vi "config_test2.vi"() -> ()   [LabVIEW 2015]
uses:
  <vilib>/Utility/Data Type/NI_Data Type.lvlib
  <vilib>/Utility/config.llb/NI_LVConfig.lvlib
  <vilib>/Utility/config.llb/Write Key (I32).vi
  <vilib>/Utility/config.llb/Write Key (String).vi
  <vilib>/Utility/config.llb/Write Key (Double).vi
panel:
  in  "Tab Control":enum32{"Page 1", "Page 2"}(tab)
  in  "x":dbl
  in  "y":dbl
  out "x+y":dbl
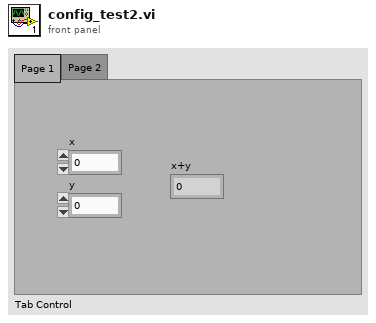
[diagram p1: front panel]
types:
  T1 = typedef "NI_LVConfig.lvlib/Config Data RefNum.ctl" = refnum<k1>
  T2 = typedef "NI_Data Type.lvlib/Data Type.ctl" = enum8{"Invalid Type", "Void", "I8", "I16", "I32", "I64", "U8", "U16", "U32", "U64", "Single Float", "Double Float", "Extended Float", "Single Complex", "Double Complex", "Extended Complex", "Enum U8", "Enum U16", "Enum U32", "Enum U64", "Single Float With Unit", "Double Float With Unit", "Extended Float With Unit", "Single Complex with Unit", "Double Complex with Unit", "Extended Complex with Unit", "Boolean", "String", "Path", "Picture", "Tag", "Array", "Cluster", "Variant", "LV Variant", "Waveform", "Timestamp", "Digital Waveform", "Digital Data", "ExpressData", "Refnum", "External Data", "VI", "Poly VI", "LabVIEW Class Instance", "Fixed Point"}
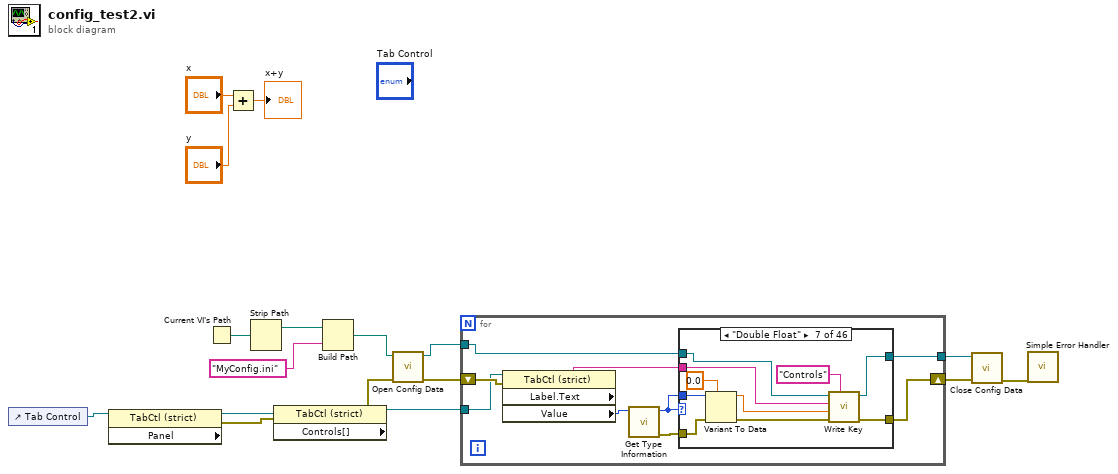
[diagram p0: block diagram]
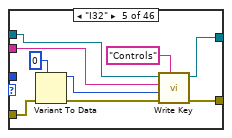
[diagram p6: hidden frame]
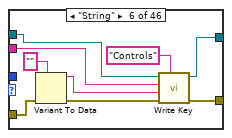
[diagram p7: hidden frame]
diagram:
  n1 = control-ref of="Tab Control"() -> (w14:refnum<vi>)
  n2 = property class="TabCtl (strict)" props=["Panel"](reference=w14) -> (reference out=w2:refnum<vi>, error out=w13:errorcluster)  [unwired: 1 in, 1 out]
  n3 = Current VI's Path() -> (path=w12:path)
  n4 = Add(x="x", y="y") -> (x+y=→"x+y":dbl)
  n5 = Strip Path(path=w12) -> (stripped path=w11:path)  [unwired: 1 out]
  n6 = property class="TabCtl (strict)" props=["Controls[]"](reference=w2, error in=w13) -> (reference out=w1:refnum<vi>, error out=w4:errorcluster)  [unwired: 1 out]
  n7 = Build Path(base path=w11, name or relative path="MyConfig.ini") -> (appended path=w9:path)
  n8 = call <vilib>:"Open Config Data.vi"("error in (no error)"=w4, "configuration file path"=w9) -> ("error out"=w3:errorcluster, "refnum"=w8:T1)  [unwired: 7 in, 1 out]
  n9 = for {
    tunnel: w8 -> [w22]
    shift-right: [w20] -> w6
    shift-left: w3 -> [w26]
    tunnel: [w21] -> w7
    tunnel: w1 -> [w19]
    n10 = property class="TabCtl (strict)"(reference=w19, error in=w26) -> ("Label.Text"=w23:string, "Value"=w24:enum32{"Page 1", "Page 2"})  [unwired: 2 out]
    n11 = call <vilib>:"Get Type Information.vi"("Variant"=w24) -> ("error out"=w25:errorcluster, "Type"=w18:T2)  [unwired: 6 in, 3 out]
    n12 = case shown="\"Double Float\"" w18 {
      tunnel: w25 -> [w27 w29 w31 w33 w43 w52 w62 w63 w65 w67 w69 w71 w73 w75 w77 w79 w81 w83 w85 w87 w89 w91 w93 w95 w97 w99 w101 w103 w105 w107 w109 w111 w113 w115 w117 w119 w121 w123 w125 w127 w129 w131 w133 w135 w137 w139]
      tunnel: w23 -> [_ _ _ _ w40 w49 w59 _ _ _ _ _ _ _ _ _ _ _ _ _ _ _ _ _ _ _ _ _ _ _ _ _ _ _ _ _ _ _ _ _ _ _ _ _ _ _]
      tunnel: w22 -> [w28 w30 w32 w34 w39 w48 w58 w64 w66 w68 w70 w72 w74 w76 w78 w80 w82 w84 w86 w88 w90 w92 w94 w96 w98 w100 w102 w104 w106 w108 w110 w112 w114 w116 w118 w120 w122 w124 w126 w128 w130 w132 w134 w136 w138 w140]
      tunnel: [w28 w30 w32 w34 w37 w46 w56 w64 w66 w68 w70 w72 w74 w76 w78 w80 w82 w84 w86 w88 w90 w92 w94 w96 w98 w100 w102 w104 w106 w108 w110 w112 w114 w116 w118 w120 w122 w124 w126 w128 w130 w132 w134 w136 w138 w140] -> w21
      tunnel: [w27 w29 w31 w33 w36 w45 w55 w63 w65 w67 w69 w71 w73 w75 w77 w79 w81 w83 w85 w87 w89 w91 w93 w95 w97 w99 w101 w103 w105 w107 w109 w111 w113 w115 w117 w119 w121 w123 w125 w127 w129 w131 w133 w135 w137 w139] -> w20
      tunnel: w18 -> [_ _ _ _ _ _ w53 _ _ _ _ _ _ _ _ _ _ _ _ _ _ _ _ _ _ _ _ _ _ _ _ _ _ _ _ _ _ _ _ _ _ _ _ _ _ _]
      frame "Invalid Type", Default {
      }
      frame "Void" {
      }
      frame "I8" {
      }
      frame "I16" {
      }
      frame "I32" {
        n13 = Variant To Data(error in=w43, type=0) -> (data=w41:i32, error out=w42:errorcluster)  [unwired: 1 in]
        n14 = call-poly <vilib>:"Write Key.vi"("section"="Controls", "error in (no error)"=w42, "value"=w41, "key"=w40, "refnum"=w39) -> ("error out"=w36:errorcluster, "refnum out"=w37:T1)  [unwired: 4 in, 1 out]
      }
      frame "String" {
        n15 = Variant To Data(error in=w52, type="") -> (data=w50:string, error out=w51:errorcluster)  [unwired: 1 in]
        n16 = call-poly <vilib>:"Write Key.vi"("section"="Controls", "error in (no error)"=w51, "value"=w50, "key"=w49, "refnum"=w48) -> ("error out"=w45:errorcluster, "refnum out"=w46:T1)  [unwired: 4 in, 1 out]
      }
      frame "Double Float" {
        n17 = Variant To Data(error in=w62, type=0.0, Variant=w53) -> (data=w60:dbl, error out=w61:errorcluster)
        n18 = call-poly <vilib>:"Write Key.vi"("section"="Controls", "error in (no error)"=w61, "value"=w60, "key"=w59, "refnum"=w58) -> ("error out"=w55:errorcluster, "refnum out"=w56:T1)  [unwired: 4 in, 1 out]
      }
      frame "I64" {
      }
      frame "U8" {
      }
      frame "U16" {
      }
      frame "U32" {
      }
      frame "U64" {
      }
      frame "Single Float" {
      }
      frame "Extended Float" {
      }
      frame "Single Complex" {
      }
      frame "Double Complex" {
      }
      frame "Extended Complex" {
      }
      frame "Enum U8" {
      }
      frame "Enum U16" {
      }
      frame "Enum U32" {
      }
      frame "Enum U64" {
      }
      frame "Single Float With Unit" {
      }
      frame "Double Float With Unit" {
      }
      frame "Extended Float With Unit" {
      }
      frame "Single Complex with Unit" {
      }
      frame "Double Complex with Unit" {
      }
      frame "Extended Complex with Unit" {
      }
      frame "Boolean" {
      }
      frame "Path" {
      }
      frame "Picture" {
      }
      frame "Tag" {
      }
      frame "Array" {
      }
      frame "Cluster" {
      }
      frame "Variant" {
      }
      frame "LV Variant" {
      }
      frame "Waveform" {
      }
      frame "Timestamp" {
      }
      frame "Digital Waveform" {
      }
      frame "Digital Data" {
      }
      frame "ExpressData" {
      }
      frame "Refnum" {
      }
      frame "External Data" {
      }
      frame "VI" {
      }
      frame "Poly VI" {
      }
      frame "LabVIEW Class Instance" {
      }
      frame "Fixed Point" {
      }
    }
  }
  n19 = call <vilib>:"Close Config Data.vi"("error in (no error)"=w6, "refnum"=w7) -> ("error out"=w5:errorcluster)  [unwired: 8 in, 1 out]
  n20 = call <vilib>:"Simple Error Handler.vi"("error in (no error)"=w5) -> ()  [unwired: 4 in, 5 out]
